vi "CalcPulsePrams.vi"(9 "Digitizer Settings":T1={"Digitizer delay (us) "=0.0, "rf points per line"=2048, "lines per plane"=128, "Samp Rate (Hz)"=100000000.0, "Additional dig delay (us)"=0.0, "Voltage Scale"=0.4, "Pre-Looks"=0, "Offset delay (us)"=0.0, "bits A/D"=8, "Avg Num"=1, "DigTimeOut"=5.0, "Rel Dig Delay"=0.0, "Dig Ch"=0, "LeCroyCluster"={"LeCroy Channels"=[TRUE, FALSE, FALSE, FALSE], "LC read pt offset"=0.0, "Sweep Avg"=FALSE}, "Main Digitizer"=enum."NI Digitizer", "Dig Config"=enum."Single channel", "Digitizer ID Cluster"={"Acqiris/Alazar/SP ID"=[], "NI Instr Handles"=[], "LeCroy VISA"="", "GaGe Handle"={"Handle"=0, "Sample size"=0, "Resolution"=0, "Offset"=0, "Channels"=0, "Boards"=0}, "ATS Ref"="ATS9350", "Acqiris Address"=["PCI::INSTR0"], "ADQRef"=refnum, "adq_cu_ptr"=refnum}, "Trigger Settings"={"Trig Source"=1, "Trig Coupling"=0, "Trig Slope"=0, "Level (mV)"=1500.0}, "Bulk Acq"=FALSE, "Bulk Start Indexes"=[], "Data Ref RF"=refnum, "NI ID/Channel"=[], "Total Dig CH"=5, "Xtra Ann Trig delay (us)"=10.0, "Fix Z Delay?"=FALSE, "One Way Transmission?"=FALSE, "Data Ref Log"=refnum} {"Trigger Settings"."Trig Slope" items=["Positive", "Negative"]; "Trigger Settings"."Level (mV)" format="%.2f"; "Trigger Settings"."Trig Coupling" items=["DC 1 MOhm", "AC 1 MOhm", "DC 50 Ohm", "AC 50 Ohm"]; "Trigger Settings"."Trig Source" items=["Chan 1", "External"]; "Rel Dig Delay" format="%.2f"; "DigTimeOut" format="%.2f"; "Avg Num" min=1; "Offset delay (us)" format="%.2f"; "Additional dig delay (us)" format="%.2f"; "Digitizer delay (us)" format="%.2f"}, 10 "Array":sgl[][][](array[numeric]), 11 "Pressure Cal Parameters":T6={"Center Freq (MHz)"=0.0, "PRF (kHz)"=1.0, "Pulse window (us)"=0.0, "Hydrophone"=enum."PAL #1048", "booster amp?"=TRUE} {"Pulse window (us)" format="%.2f"; "PRF (kHz)" format="%.2f"; "Center Freq (MHz)" format="%.2f"}) -> (3 "Data":T5(array[cluster]) {"pos peak pressure (MPa)" format="%.2f"})   [LabVIEW 2022 SP3]
uses:
  HydrophoneSettings.ctl
  Hydros.ctl
  ScanningControl/Digitizers/-DigitizerRoutines/DigitizerSettings.ctl
  ScanningControl/Digitizers/-DigitizerRoutines/Digitizer.ctl
  ScanningControl/Digitizers/-DigitizerRoutines/DigConfig.ctl
  ScanningControl/Digitizers/-DigitizerRoutines/DigitizerID.ctl
  C:/Windows/System32/ADQAPI_dotNet_helper.dll
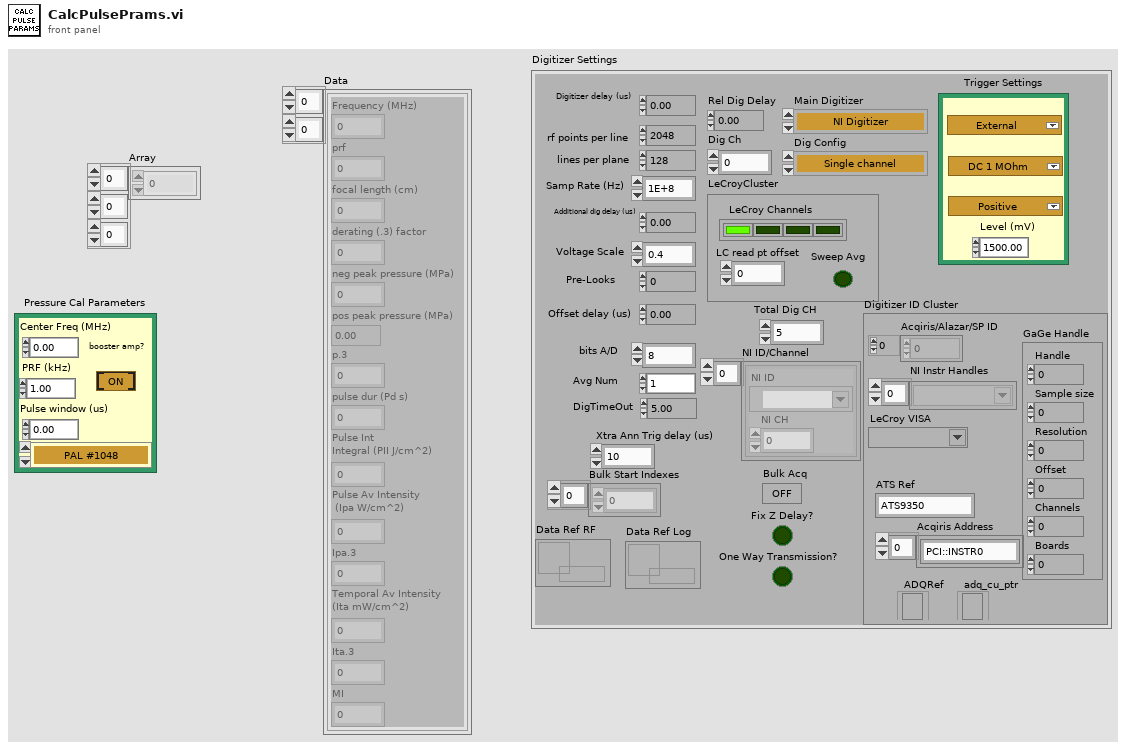
[diagram p1: front panel]
types:
  T1 = typedef "DigitizerSettings.ctl" = cluster{"Digitizer delay (us) ":dbl, "rf points per line":i32, "lines per plane":i32, "Samp Rate (Hz)":dbl, "Additional dig delay (us)":dbl, "Voltage Scale":dbl, "Pre-Looks":i32, "Offset delay (us)":dbl, "bits A/D":i8, "Avg Num":i32, "DigTimeOut":sgl, "Rel Dig Delay":sgl, "Dig Ch":i32, "LeCroyCluster":cluster{"LeCroy Channels":bool[], "LC read pt offset":dbl, "Sweep Avg":bool}, "Main Digitizer":T2, "Dig Config":T3, "Digitizer ID Cluster":T4, "Trigger Settings":cluster{"Trig Source":u16, "Trig Coupling":u16, "Trig Slope":u16, "Level (mV)":dbl}, "Bulk Acq":bool, "Bulk Start Indexes":i32[], "Data Ref RF":refnum<data-value>, "NI ID/Channel":cluster{"NI ID":refnum<k15>, "NI CH":i32}[], "Total Dig CH":i32, "Xtra Ann Trig delay (us)":dbl, "Fix Z Delay?":bool, "One Way Transmission?":bool, "Data Ref Log":refnum<data-value>}
  T2 = typedef "Digitizer.ctl" = enum16{"Acqiris Digitizer", "NI Digitizer", "LeCroy", "GaGe", "AlazarTech", "No Digitizer", "Teledyne"}
  T3 = typedef "DigConfig.ctl" = enum16{"Single channel", "2 Chans w/ 2 Acqiris", "2 Chans w/ 1 Acqiris", "5-CH Pulser New", "5-CH pulser w/ ann array", "5-pass style ann array", "Empty"}
  T4 = typedef "DigitizerID.ctl" = cluster{"Acqiris/Alazar/SP ID":u32[], "NI Instr Handles":refnum<k15>[], "LeCroy VISA":refnum<visa-resource-name>, "GaGe Handle":cluster{"Handle":u32, "Sample size":u32, "Resolution":i32, "Offset":i32, "Channels":u32, "Boards":u32}, "ATS Ref":string, "Acqiris Address":string[], "ADQRef":refnum<k24>, "adq_cu_ptr":refnum<k24>}
  T5 = cluster{"Frequency (MHz)":dbl, "prf":dbl, "focal length (cm)":dbl, "derating (.3) factor":dbl, "neg peak pressure (MPa)":dbl, "pos peak pressure (MPa)":dbl, "p.3":dbl, "pulse dur (Pd s)":dbl, "Pulse Int \nIntegral (PII J/cm^2)":dbl, "Pulse Av Intensity\n (Ipa W/cm^2)":dbl, "Ipa.3":dbl, "Temporal Av Intensity \n(Ita mW/cm^2)":dbl, "Ita.3":dbl, "MI":dbl}[][]
  T6 = typedef "HydrophoneSettings.ctl" = cluster{"Center Freq (MHz)":dbl, "PRF (kHz)":dbl, "Pulse window (us)":dbl, "Hydrophone":T7, "booster amp?":bool}
  T7 = typedef "Hydros.ctl" = enum16{"PAL #1048", "PAL #525", "PAL #430a", "PAL #192", "DEAD PAL # 1403", "LOST UHI Onda", "DEAD PAL #1818", "PAL #1974", "DEAD #2266 w/booster", "PAL #2524 w/booster", "PAL FP21-20T", "PAL FP160-13  ", "PAL FP141-20", "PAL FP158-08T"}
  T8 = cluster{"Frequency (MHz)":dbl, "prf":dbl, "focal length (cm)":dbl, "derating (.3) factor":dbl, "neg peak pressure (MPa)":dbl, "pos peak pressure (MPa)":dbl, "p.3":dbl, "pulse dur (Pd s)":dbl, "Pulse Int \nIntegral (PII J/cm^2)":dbl, "Pulse Av Intensity\n (Ipa W/cm^2)":dbl, "Ipa.3":dbl, "Temporal Av Intensity \n(Ita mW/cm^2)":dbl, "Ita.3":dbl, "MI":dbl}
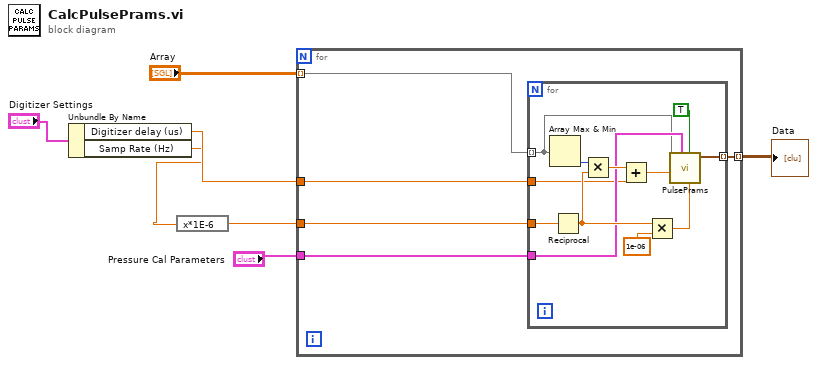
[diagram p0: block diagram]
diagram:
  n1 = Unbundle By Name("Digitizer Settings") -> ("Digitizer delay (us)"=w2:dbl, "Samp Rate (Hz)"=w1:dbl)
  n2 = expression code="x*1E-6"(w1) -> (w6:dbl)
  n3 = for {
    tunnel: "Pressure Cal Parameters" -> [w12]
    tunnel: [w11] -> w4 mode=indexing
    tunnel: w6 -> [w10]
    tunnel: w2 -> [w9]
    tunnel: "Array" -> [w8] mode=indexing
    n4 = for {
      tunnel: w12 -> [w19]
      tunnel: w8 -> [w18] mode=indexing
      tunnel: [w17] -> w11 mode=indexing
      tunnel: w10 -> [w16]
      tunnel: w9 -> [w15]
      n5 = Array Max & Min(array=w18) -> (min index (indices)=w21:i32)  [unwired: 3 out]
      n6 = Reciprocal(x=w16) -> (1/x=w20:dbl)
      n7 = Multiply(x=w21, y=w20) -> (x*y=w24:dbl)
      n8 = Add(x=w24, y=w15) -> (x+y=w23:dbl)
      n9 = Multiply(x=w20, y=1e-06) -> (x*y=w14:dbl)
      n10 = call "PulsePrams.vi"("sample rate (s/Pt)"=w14, "Compute window?"=TRUE, "Pressure Cal Parameters"=w19, "delay (ms)"=w23, "Data"=w18) -> ("Pulse Parameters"=w17:T8)  [unwired: 2 in, 4 out]
    }
  }
  "Data" <- w4
